vi "to UINT32.vi"(8 "error in":errorcluster, 11 "byte":u8[](array[numeric]) format="%b") -> (0 "error out":errorcluster, 3 "UINT32":u32)   [LabVIEW 2020, in "wamplv.lvlib" / "MessagePack.lvclass"]
uses:
  MessagePack.lvclass
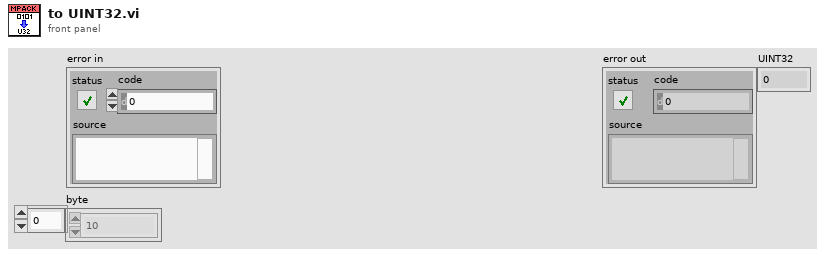
[diagram p1: front panel]
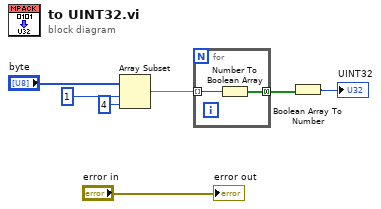
[diagram p0: block diagram]
diagram:
  n1 = Array Subset(array="byte", index=1, length=4) -> (w3:u8[])
  n2 = for {
    tunnel: w3 -> [w9] mode=indexing
    tunnel: [w8] -> w2 mode=concatenating
    n3 = Number To Boolean Array(number=w9) -> (Boolean array=w8:bool[])
  }
  n4 = Boolean Array To Number(Boolean array=w2) -> (number=→"UINT32":u32)
  "error out" <- "error in"
